vi "Stage 3.2 Getting the GUI out.vi"() -> ()   [LabVIEW 2020]
uses:
  HRM-User_events.ctl
  <vilib>/measure/matone.llb/Extract Single Tone Information 1 Chan.vi
  <vilib>/measure/NI_MAPro.lvlib
panel:
  out "error out":errorcluster
  out "raw data":waveform(dbl)
  out "error out Hardware":errorcluster
  in  "Addition signal to remove (0) [s]":dbl
  out "Pulse":dbl
  out "Filtered":waveform(dbl)(graph)
  in  "Samples size (10) [s]":i32=10
  out "unfiltered wf":waveform(dbl)(graph)
  in  "Stop":bool
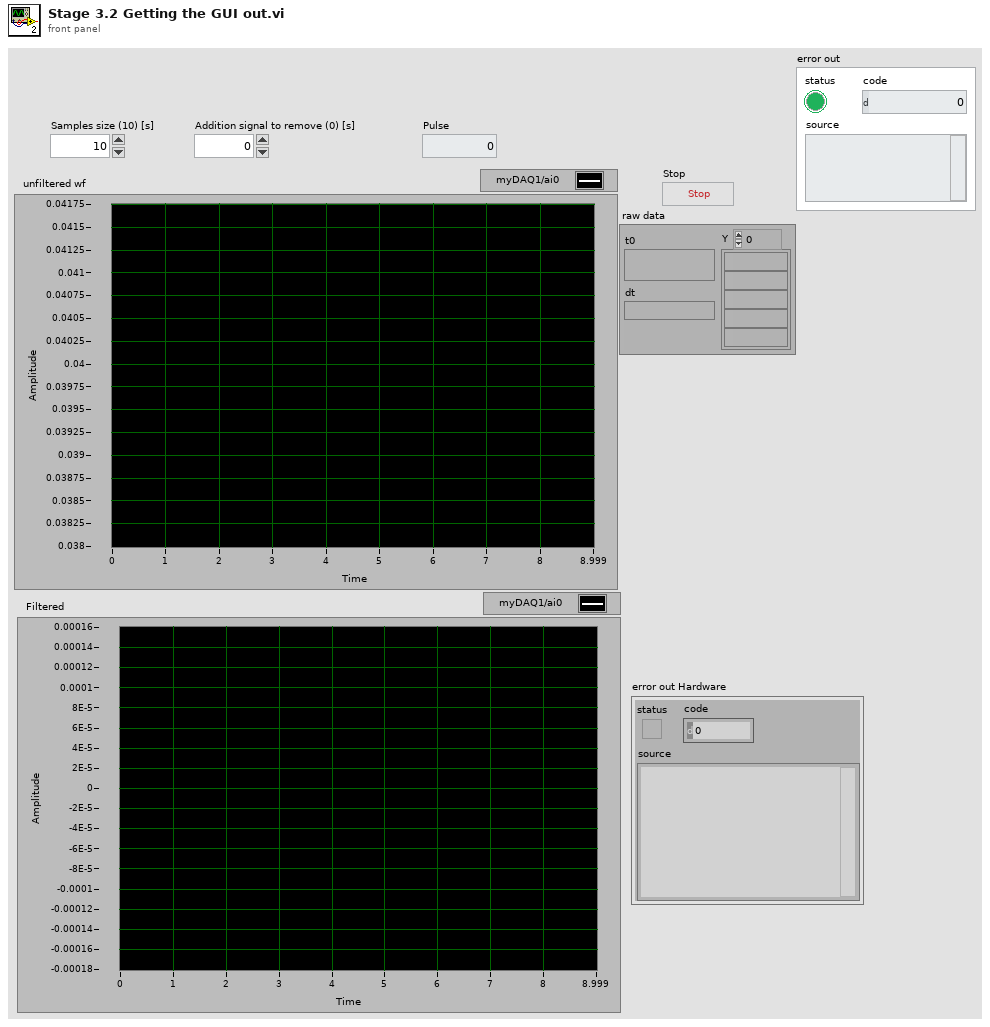
[diagram p1: front panel]
types:
  T1 = typedef "HRM-User_events.ctl" = cluster{"Signal to remove":refnum<user-event>, "Sample size":refnum<user-event>, "Filtered wf":refnum<user-event>, "Unfiltered wf":refnum<user-event>, "Raw wf":refnum<user-event>, "Pulse":refnum<user-event>}
  T2 = cluster{"Samples size (10)":i32, "Addition signal to remove":dbl, "Unfiltered wf":waveform(dbl), "User events":T1}
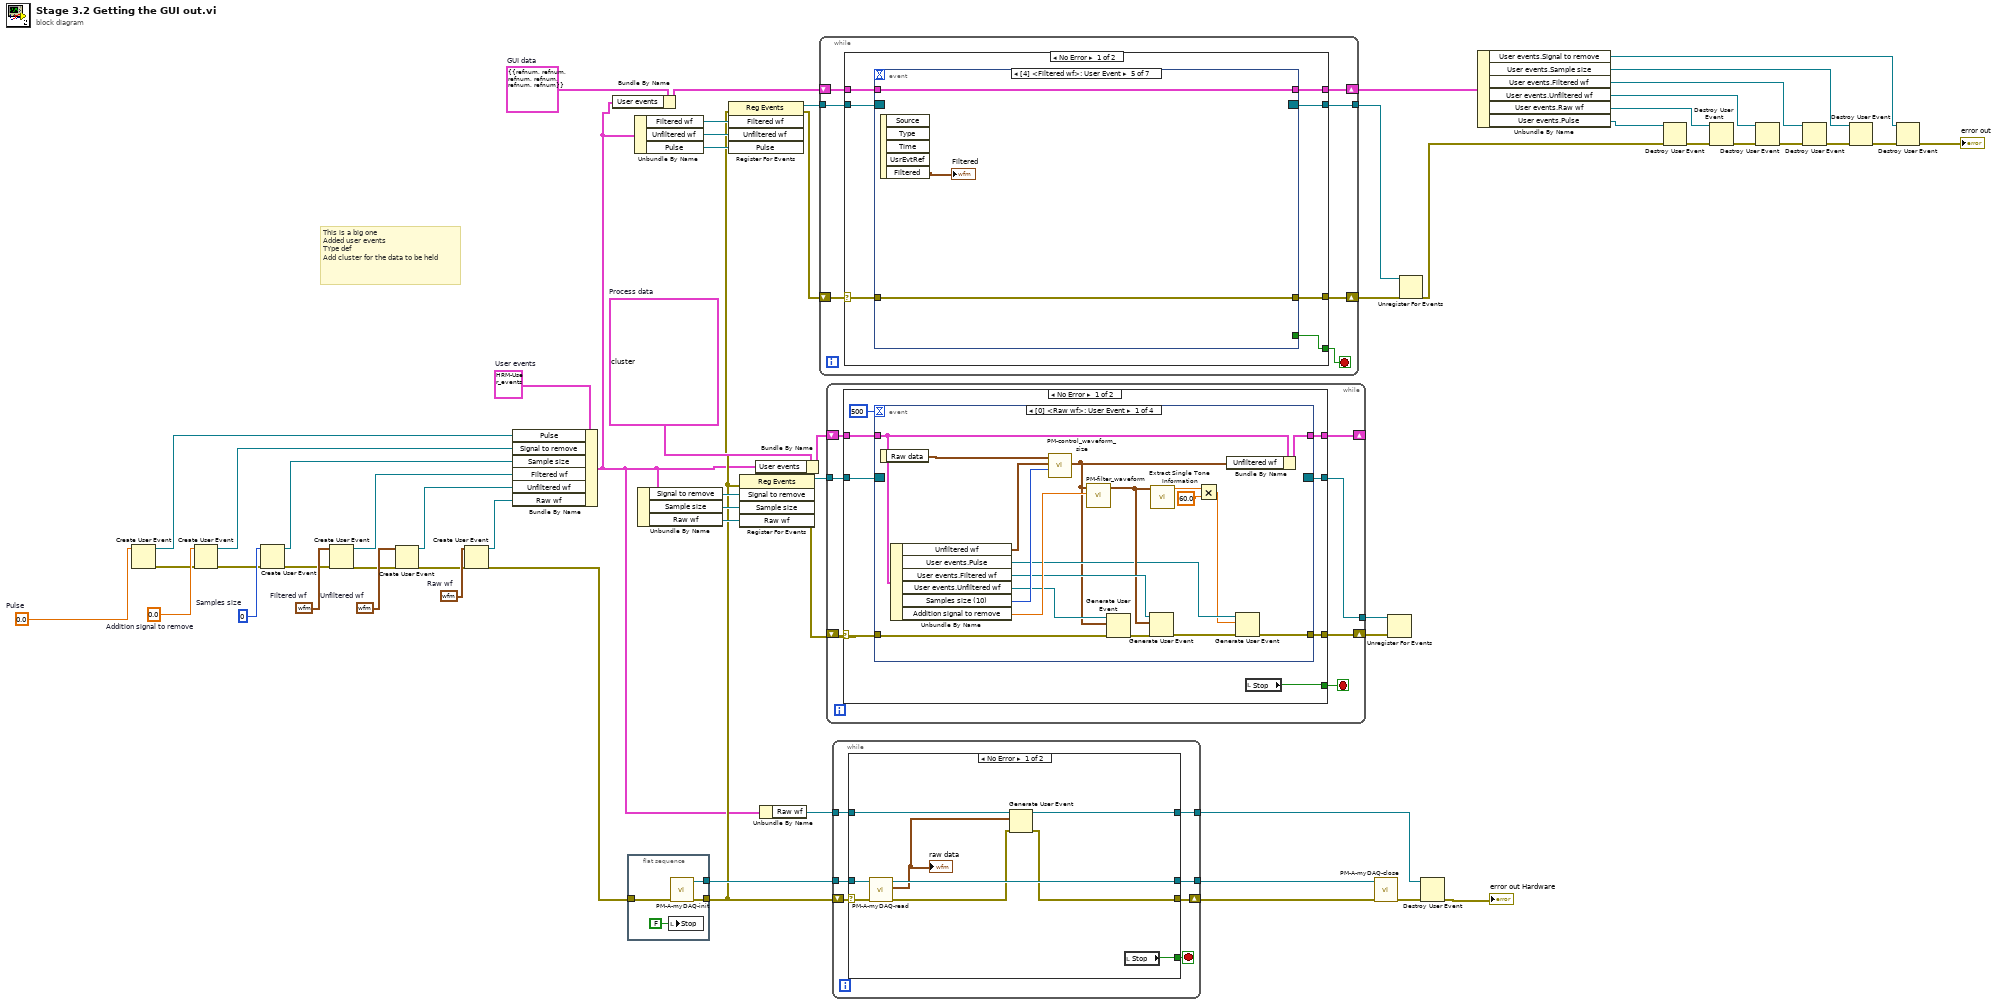
[diagram p0: block diagram]
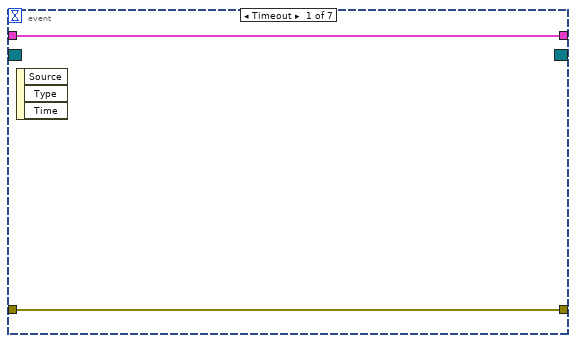
[diagram p2: hidden frame]
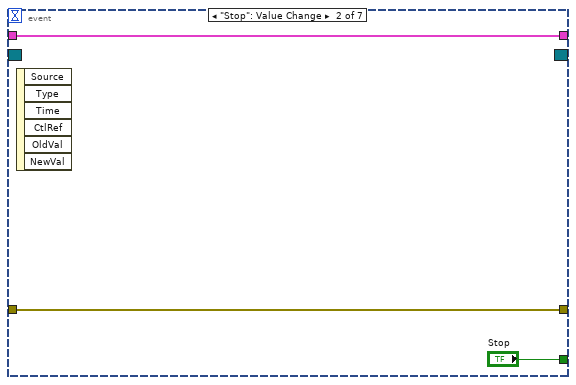
[diagram p3: hidden frame]
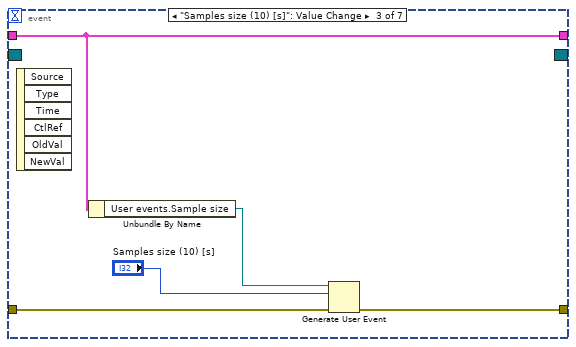
[diagram p4: hidden frame]
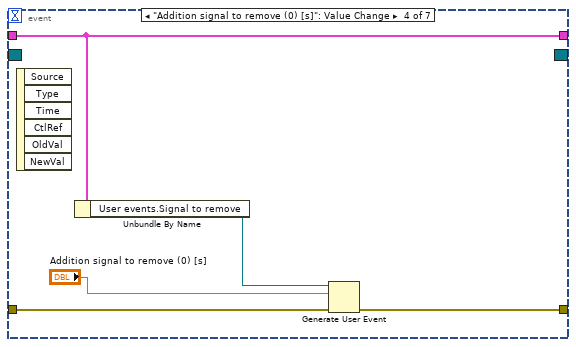
[diagram p5: hidden frame]
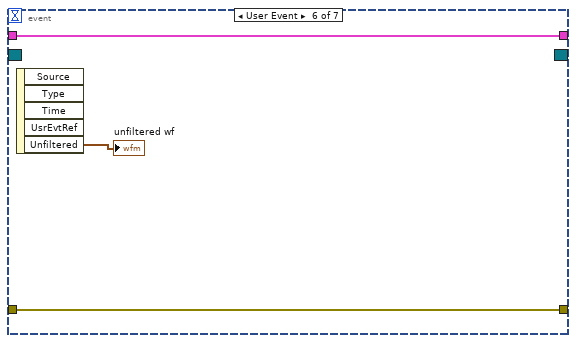
[diagram p6: hidden frame]
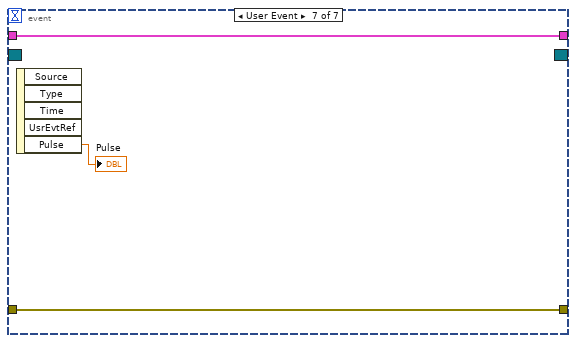
[diagram p7: hidden frame]
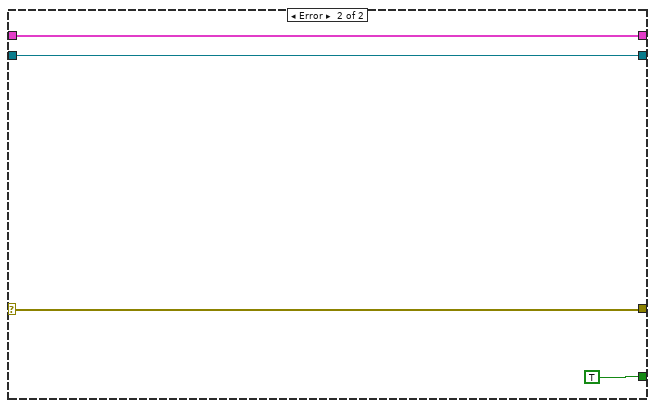
[diagram p8: hidden frame]
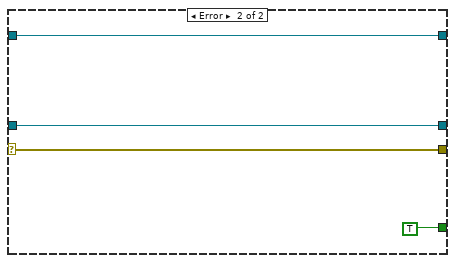
[diagram p9: hidden frame]
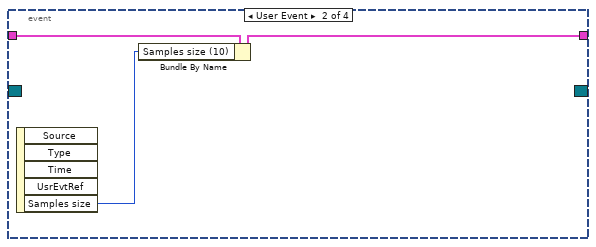
[diagram p10: hidden frame]
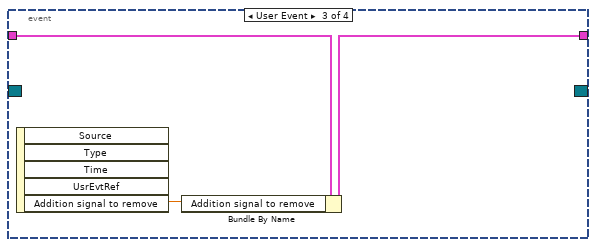
[diagram p11: hidden frame]
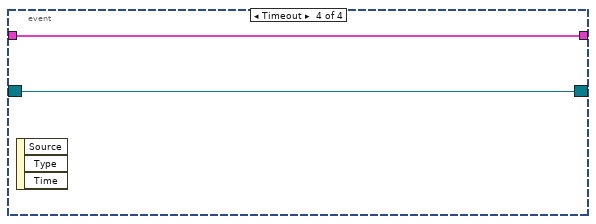
[diagram p12: hidden frame]
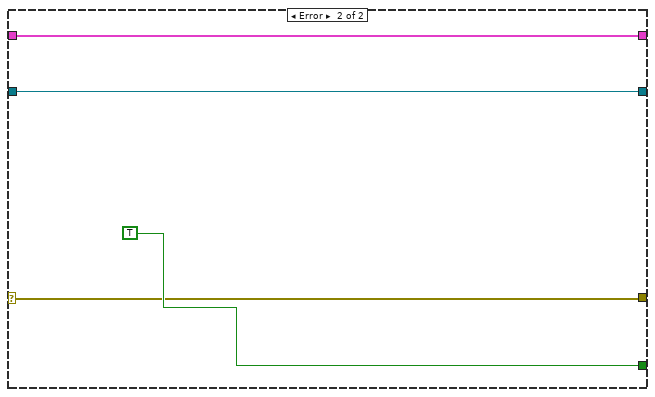
[diagram p13: hidden frame]
diagram:
  w22 = cluster{"User events":T1} {"User events"={"Signal to remove"=refnum, "Sample size"=refnum, "Filtered wf"=refnum, "Unfiltered wf"=refnum, "Raw wf"=refnum, "Pulse"=refnum}}  # GUI data
  w30 = 0.0  # Pulse
  w41 = T1 {"Signal to remove"=refnum, "Sample size"=refnum, "Filtered wf"=refnum, "Unfiltered wf"=refnum, "Raw wf"=refnum, "Pulse"=refnum}  # User events
  w42 = T2 {"Samples size (10)"=10, "Addition signal to remove"=0.0, "Unfiltered wf"={"t0"=timestamp(0 s since 1904-01-01), "dt"=1.0, "Y"=[]}, "User events"={"Signal to remove"=refnum, "Sample size"=refnum, "Filtered wf"=refnum, "Unfiltered wf"=refnum, "Raw wf"=refnum, "Pulse"=refnum}}  # Process data
  w47 = 0  # Samples size
  w48 = 0.0  # Addition signal to remove
  w49 = waveform(dbl) {"t0"=timestamp(0 s since 1904-01-01), "dt"=1.0, "Y"=[]}  # Filtered wf
  w50 = waveform(dbl) {"t0"=timestamp(0 s since 1904-01-01), "dt"=1.0, "Y"=[]}  # Unfiltered wf
  w57 = waveform(dbl) {"t0"=timestamp(0 s since 1904-01-01), "dt"=1.0, "Y"=[]}  # Raw wf
  # "This is a big one\nAdded user events\nTYpe def\nAdd cluster for the data to be held"
  n1 = Create User Event(user event datatype=w30) -> (user event=w29:refnum<user-event>, error out=w28:errorcluster)  [unwired: 1 in]
  n2 = Create User Event(user event datatype=w48, error in=w28) -> (user event=w40:refnum<user-event>, error out=w43:errorcluster)
  n3 = Create User Event(user event datatype=w47, error in=w43) -> (user event=w39:refnum<user-event>, error out=w44:errorcluster)
  n4 = Create User Event(user event datatype=w49, error in=w44) -> (user event=w38:refnum<user-event>, error out=w45:errorcluster)
  n5 = Create User Event(user event datatype=w50, error in=w45) -> (user event=w37:refnum<user-event>, error out=w46:errorcluster)
  n6 = Create User Event(user event datatype=w57, error in=w46) -> (user event=w36:refnum<user-event>, error out=w56:errorcluster)
  n7 = Bundle By Name(cluster=w41, "Pulse"=w29, "Signal to remove"=w40, "Sample size"=w39, "Filtered wf"=w38, "Unfiltered wf"=w37, "Raw wf"=w36) -> (w1:T1)
  n8 = Bundle By Name(cluster=w22, "User events"=w1) -> (w2:cluster{"User events":T1})
  n9 = flat-sequence {
    tunnel: [w64] -> w58
    tunnel: [w63] -> w23
    tunnel: w56 -> [w61]
    frame #0 {
      n10 = local write "Stop"(FALSE ("Stop")) -> ()
      n11 = call "PM-A-myDAQ-init.vi"("error in"=w61) -> ("error out"=w63:errorcluster, "Refnum out"=w64:refnum<k21>)  [unwired: 9 in]
    }
  }
  n12 = Unbundle By Name(w1) -> ("Filtered wf"=w26:refnum<user-event>, "Unfiltered wf"=w25:refnum<user-event>, "Pulse"=w24:refnum<user-event>)
  n13 = Unbundle By Name(w1) -> ("Signal to remove"=w35:refnum<user-event>, "Sample size"=w34:refnum<user-event>, "Raw wf"=w32:refnum<user-event>)
  n14 = register-events(error in=w23, w26, w25, w24) -> (reference out=w27:refnum<event-registration>, error out=w21:errorcluster)  [unwired: 1 in]
  n15 = register-events(error in=w23, w35, w34, w32) -> (reference out=w51:refnum<event-registration>, error out=w52:errorcluster)  [unwired: 1 in]
  n16 = Bundle By Name(cluster=w42, "User events"=w1) -> (w31:T2)
  n17 = Unbundle By Name(w1) -> ("Raw wf"=w33:refnum<user-event>)
  n18 = while {
    tunnel: w27 -> [w71]
    shift-right: [w67] -> w19
    shift-left: w21 -> [w68]
    shift-right: [w66] -> w16
    shift-left: w2 -> [w70]
    tunnel: [w65] -> w20
    stop <- w69 stop-if-true
    n19 = case shown="No Error" w68 {
      selector: w68 -> [w75 w105]
      tunnel: [w76 TRUE ("Stop")] -> w69
      tunnel: [w74 w105] -> w67
      tunnel: w71 -> [w78 w103]
      tunnel: w70 -> [w77 w104]
      tunnel: [w73 w104] -> w66
      tunnel: [w72 w103] -> w65
      frame No Error {
        n20 = event shown="[4] <Filtered wf>: User Event" {
          selector: w78 -> [_ _ _ _ _ _ _]
          dyn-events: [_ _ _ _ _ _ _] -> w72
          timeout: _ -> [_ _ _ _ _ _ _]
          tunnel: w77 -> [w80 w81 w86 w91 w95 w98 w101]
          tunnel: [_ "Stop" _ _ _ _ _] -> w76
          tunnel: [w79 w82 w87 w92 w96 w99 w102] -> w74
          tunnel: w75 -> [w79 w82 w88 w93 w96 w99 w102]
          tunnel: [w80 w81 w86 w91 w95 w98 w101] -> w73
          event Timeout {
            n21 = event-data() -> ()  [unwired: 1 in, 3 out]
          }
          event "Stop": Value Change {
            n22 = event-data() -> ()  [unwired: 1 in, 6 out]
          }
          event "Samples size (10) [s]": Value Change {
            n23 = event-data() -> ()  [unwired: 1 in, 6 out]
            n24 = Unbundle By Name(w86) -> ("User events.Sample size"=w85:refnum<user-event>)
            n25 = Generate User Event(user event=w85, event data cluster="Samples size (10) [s]", error in=w88) -> (error out=w87:errorcluster)  [unwired: 1 in, 1 out]
          }
          event "Addition signal to remove (0) [s]": Value Change {
            n26 = event-data() -> ()  [unwired: 1 in, 6 out]
            n27 = Unbundle By Name(w91) -> ("User events.Signal to remove"=w90:refnum<user-event>)
            n28 = Generate User Event(user event=w90, event data cluster="Addition signal to remove (0) [s]", error in=w93) -> (error out=w92:errorcluster)  [unwired: 1 in, 1 out]
          }
          event User Event {
            n29 = event-data() -> ("Filtered"=→"Filtered":waveform(dbl))  [unwired: 1 in, 4 out]
          }
          event User Event {
            n30 = event-data() -> ("Unfiltered"=→"unfiltered wf":waveform(dbl))  [unwired: 1 in, 4 out]
          }
          event User Event {
            n31 = event-data() -> ("Pulse"=→"Pulse":dbl)  [unwired: 1 in, 4 out]
          }
        }
      }
      frame Error {
      }
    }
  }
  n32 = while {
    tunnel: w51 -> [w111]
    shift-right: [w109] -> _
    shift-left: w31 -> [w110]
    shift-right: [w108] -> w18
    shift-left: w52 -> [w112]
    tunnel: [w107] -> w17
    stop <- w113 stop-if-true
    n33 = case shown="No Error" w112 {
      selector: w112 -> [w118 w149]
      tunnel: [w116 TRUE ("Stop")] -> w113
      tunnel: w111 -> [w121 w148]
      tunnel: w110 -> [w120 w150]
      tunnel: [w119 w150] -> w109
      tunnel: [w117 w149] -> w108
      tunnel: [w114 w148] -> w107
      frame No Error {
        n34 = event shown="[0] <Raw wf>: User Event" {
          selector: w121 -> [_ _ _ w146]
          dyn-events: [_ _ _ w146] -> w114
          timeout: 500 -> [_ _ _ _]
          tunnel: w120 -> [w137 w142 w145 w147]
          tunnel: [w126 w141 w144 w147] -> w119
          tunnel: w118 -> [w123 _ _ _]
          tunnel: [w122 _ _ _] -> w117
          event User Event {
            n35 = event-data() -> ("Raw data"=w138:waveform(dbl))  [unwired: 1 in]
            n36 = Unbundle By Name(w137) -> ("Unfiltered wf"=w124:waveform(dbl), "User events.Pulse"=w129:refnum<user-event>, "User events.Filtered wf"=w132:refnum<user-event>, "User events.Unfiltered wf"=w134:refnum<user-event>, "Samples size (10)"=w136:i32, "Addition signal to remove"=w135:dbl)
            n37 = call "PM-control_waveform_size.vi"("Samples s"=w136, "old waveform"=w124, "New waveform"=w138) -> ("waveform"=w125:waveform(dbl))  [unwired: 8 in]
            n38 = call "PM-filter_waveform.vi"("Addition signal to remove (0) [s]"=w135, "waveform in"=w125) -> ("waveform out"=w131:waveform(dbl))  [unwired: 8 in, 1 out]
            n39 = Generate User Event(user event=w134, event data cluster=w125, error in=w123) -> (error out=w133:errorcluster)  [unwired: 1 in, 1 out]
            n40 = Generate User Event(user event=w132, event data cluster=w131, error in=w133) -> (error out=w130:errorcluster)  [unwired: 1 in, 1 out]
            n41 = call-poly <vilib>:"Extract Single Tone Information.vi"("time signal in"=w131) -> ("detected frequency"=w128:dbl)  [unwired: 5 in, 5 out]
            n42 = Multiply(x=w128, y=60.0) -> (x*y=w127:dbl)
            n43 = Bundle By Name(cluster=w137, "Unfiltered wf"=w125) -> (w126:T2)
            n44 = Generate User Event(user event=w129, event data cluster=w127, error in=w130) -> (error out=w122:errorcluster)  [unwired: 1 in, 1 out]
          }
          event User Event {
            n45 = event-data() -> ("Samples size"=w140:i32)  [unwired: 1 in, 4 out]
            n46 = Bundle By Name(cluster=w142, "Samples size (10)"=w140) -> (w141:T2)
          }
          event User Event {
            n47 = event-data() -> ("Addition signal to remove"=w143:dbl)  [unwired: 1 in, 4 out]
            n48 = Bundle By Name(cluster=w145, "Addition signal to remove"=w143) -> (w144:T2)
          }
          event Timeout {
            n49 = event-data() -> ()  [unwired: 1 in, 3 out]
          }
        }
        n50 = local read "Stop"() -> (w116:bool)
      }
      frame Error {
      }
    }
  }
  n51 = while {
    tunnel: w58 -> [w158]
    tunnel: [w156] -> w59
    shift-right: [w155] -> w60
    shift-left: w23 -> [w157]
    tunnel: w33 -> [w153]
    tunnel: [w152] -> w53
    stop <- w154 stop-if-true
    n52 = case shown="No Error" w157 {
      selector: w157 -> [w166 w170]
      tunnel: w158 -> [w167 w169]
      tunnel: [w165 w169] -> w156
      tunnel: [w160 w170] -> w155
      tunnel: [w164 TRUE ("Stop")] -> w154
      tunnel: w153 -> [w163 w168]
      tunnel: [w159 w168] -> w152
      frame No Error {
        n53 = call "PM-A-myDAQ-read.vi"("error in (no error)"=w166, "Refnum in"=w167) -> ("error out"=w161:errorcluster, "data"=w162:waveform(dbl), "Refnum out"=w165:refnum<k21>)  [unwired: 7 in]
        "raw data" <- w162
        n54 = Generate User Event(user event=w163, event data cluster=w162, error in=w161) -> (user event out=w159:refnum<user-event>, error out=w160:errorcluster)  [unwired: 1 in]
        n55 = local read "Stop"() -> (w164:bool)
      }
      frame Error {
      }
    }
  }
  n56 = call "PM-A-myDAQ-close.vi"("error in (no error)"=w60, "Refnum in"=w59) -> ("error out"=w55:errorcluster)  [unwired: 9 in]
  n57 = Unregister For Events(event registration refnum=w17, error in=w18) -> ()  [unwired: 1 out]
  n58 = Unregister For Events(event registration refnum=w20, error in=w19) -> (error out=w4:errorcluster)
  n59 = Destroy User Event(user event=w53, error in=w55) -> (error out=→"error out Hardware":errorcluster)
  n60 = Unbundle By Name(w16) -> ("User events.Signal to remove"=w5:refnum<user-event>, "User events.Sample size"=w6:refnum<user-event>, "User events.Filtered wf"=w7:refnum<user-event>, "User events.Unfiltered wf"=w8:refnum<user-event>, "User events.Raw wf"=w9:refnum<user-event>, "User events.Pulse"=w10:refnum<user-event>)
  n61 = Destroy User Event(user event=w10, error in=w4) -> (error out=w11:errorcluster)
  n62 = Destroy User Event(user event=w9, error in=w11) -> (error out=w15:errorcluster)
  n63 = Destroy User Event(user event=w8, error in=w15) -> (error out=w14:errorcluster)
  n64 = Destroy User Event(user event=w7, error in=w14) -> (error out=w13:errorcluster)
  n65 = Destroy User Event(user event=w6, error in=w13) -> (error out=w12:errorcluster)
  n66 = Destroy User Event(user event=w5, error in=w12) -> (error out=→"error out":errorcluster)
